vi "Get Column Info.vi"(8 "error in (no error)":errorcluster, 9 "Column Name Array (All)":string[](array[string]), 10 "Table Name":string, 11 "MS Access in":refnum<class "MS Access.lvclass">) -> (0 "error out":errorcluster, 2 "Column Information Array":T1(array[cluster]), 3 "MS Access out":refnum<class "MS Access.lvclass">)   [LabVIEW 2020, in "MS Access.lvclass"]
uses:
  MS Access.lvclass
  ODBC/ADODB.lvclass
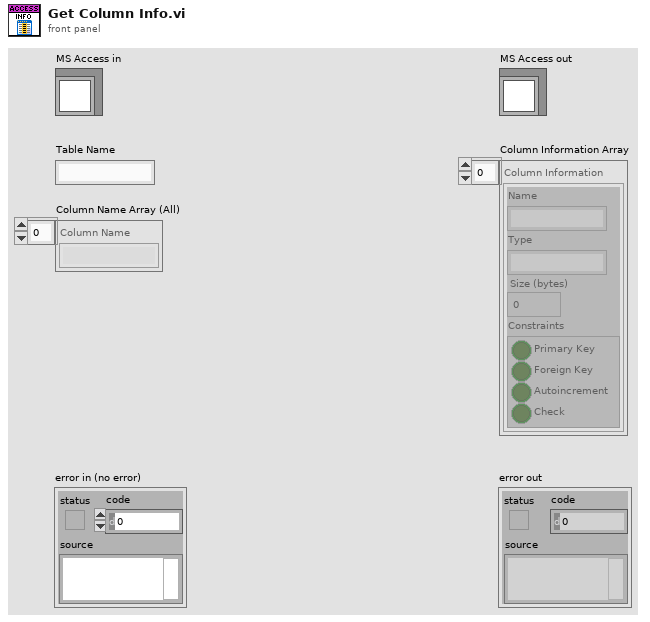
[diagram p1: front panel]
types:
  T1 = cluster{"Name":string, "Type":string, "Size (bytes)":i32, "Constraints":cluster{"Primary Key":bool, "Foreign Key":bool, "Autoincrement":bool, "Check":bool}}[]
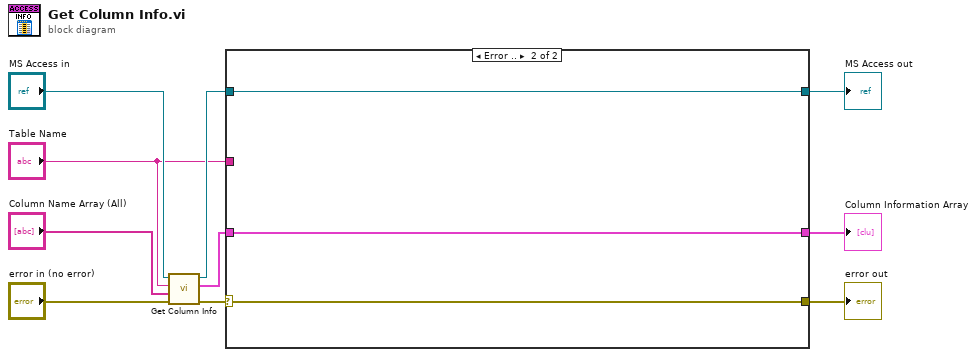
[diagram p0: block diagram]
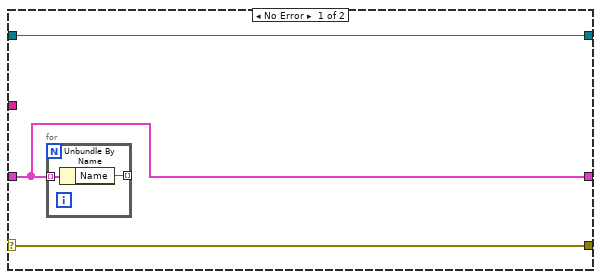
[diagram p2: hidden frame]
diagram:
  n1 = call-parent "Get Column Info.vi"("error in (no error)"="error in (no error)", "Column Name Array (All)"="Column Name Array (All)", "Table Name"="Table Name", "ODBC in"="MS Access in") -> ("error out"=w7:errorcluster, "Column Information Array"=w3:T1, "ODBC out"=w5:refnum<class "MS Access.lvclass">)  [unwired: 5 in]
  n2 = case shown="Error .." w7 {
    selector: w7 -> [w13 w18]
    tunnel: [w13 w18] -> w6
    tunnel: w5 -> [w11 w16]
    tunnel: "Table Name" -> [_ _]
    tunnel: w3 -> [w12 w17]
    tunnel: [w12 w17] -> w2
    tunnel: [w11 w16] -> w1
    frame No Error {
      n3 = for {
        tunnel: w12 -> [w15] mode=indexing
        tunnel: [w14] -> _ mode=indexing
        n4 = Unbundle By Name(w15) -> ("Name"=w14:string)
      }
    }
    frame Error {
    }
  }
  "error out" <- w6
  "MS Access out" <- w1
  "Column Information Array" <- w2
